vi "Initialize.vi"(8 "error in (no error)":errorcluster, 11 "DAQ_QPT_Throlab in":refnum<class "DAQ_QPT_Throlab.lvclass">) -> (0 "error out":errorcluster, 3 "DAQ_QPT_Throlab out":refnum<class "DAQ_QPT_Throlab.lvclass">)   [LabVIEW 2020, in "DAQ_QPT_Throlab.lvlib" / "DAQ_QPT_Throlab.lvclass"]
uses:
  DAQ_QPT_Throlab.lvclass
  DAQ_QPT_Throlab.lvclass/DAQ_QPT_Throlab.ctl
  HAL Layer/Component/DAQ/DAQ/DAQ.lvclass
  Dependency/TIRF-Lock.dll
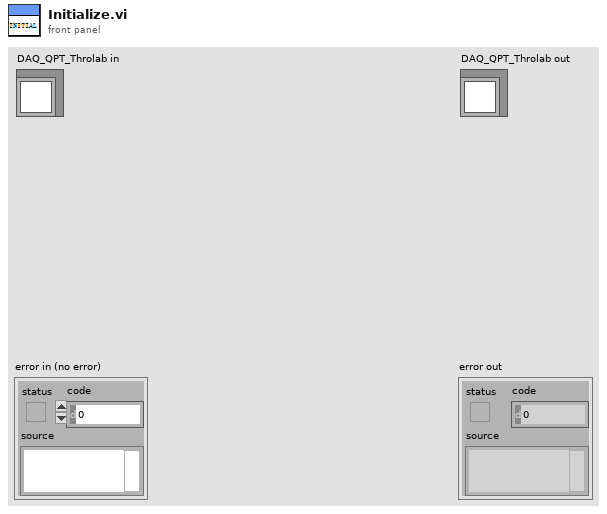
[diagram p1: front panel]
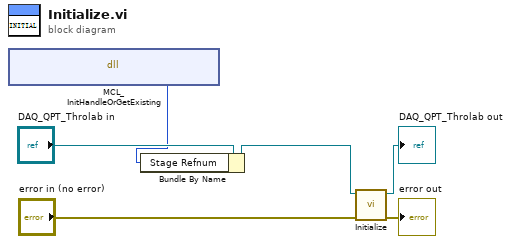
[diagram p0: block diagram]
diagram:
  n1 = dll-call lib="E:/Development/DevHardSoftware/MMicroscopyAF/Model/Real Hardware/DAQ_QPT_Throlab/Dependency/TIRF-Lock.dll" fn="MCL_InitHandleOrGetExisting" label="TIRF handle"() -> ("handle"=w1:i32)  [unwired: 3 in, 2 out]
  n2 = Bundle By Name(cluster="DAQ_QPT_Throlab in", "Stage Refnum"=w1) -> (w2:refnum<class "DAQ_QPT_Throlab.lvclass">)
  n3 = call-parent "Initialize.vi"("error in (no error)"="error in (no error)", "Device in"=w2) -> ("error out"=→"error out":errorcluster, "Device out"=→"DAQ_QPT_Throlab out":refnum<class "DAQ_QPT_Throlab.lvclass">)  [unwired: 8 in]
